vi "Draw.vi"(8 "error in (no error)":errorcluster, 10 "2D Picture in":picture, 11 "RoundRectangle in":refnum<class "RoundRectangle.lvclass">) -> (0 "error out":errorcluster, 2 "2D Picture out":picture, 3 "RoundRectangle out":refnum<class "RoundRectangle.lvclass">)   [LabVIEW 2021, in "Picture2D.lvlib" / "RoundRectangle.lvclass"]
uses:
  RoundRectangle.lvclass
  RoundRectangle.lvclass/RoundRectangle.ctl
  Rectangle/Rectangle.lvclass
  Color/Color.lvclass
  C:/Users/daal/OneDrive/LabVIEW/Class/Picture2D/Rectangle/Rectangle.lvclass
  C:/Users/daal/OneDrive/LabVIEW/Class/Picture2D/Polygone/Polygone.lvclass
  C:/Users/daal/OneDrive/LabVIEW/Class/Picture2D/Shape/Shape.lvclass
  C:/Users/daal/OneDrive/LabVIEW/Class/Picture2D/Picture2D/Picture2D.lvclass
  C:/Users/daal/OneDrive/LabVIEW/Class/Picture2D/IDrawable/IDrawable.lvclass
  C:/Users/daal/OneDrive/LabVIEW/Class/Picture2D/IMovable/IMovable.lvclass
  C:/Users/daal/OneDrive/LabVIEW/Class/Picture2D/IRotatable/IRotatable.lvclass
  C:/Users/daal/OneDrive/LabVIEW/Class/Picture2D/IScalable/IScalable.lvclass
  C:/Users/daal/OneDrive/LabVIEW/Class/Picture2D/RoundRectangle/RoundRectangle.lvclass
  Pen/Pen.lvclass
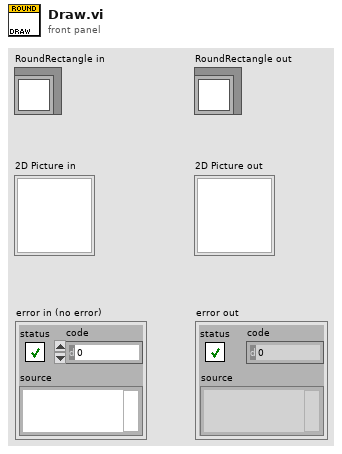
[diagram p1: front panel]
types:
  T1 = cluster{"left":i16, "top":i16, "right":i16, "bottom":i16}
  T2 = cluster{"Width":u16, "Style":enum32{"Solid", "Dash", "Dot", "DashDot", "DashDotDot"}}
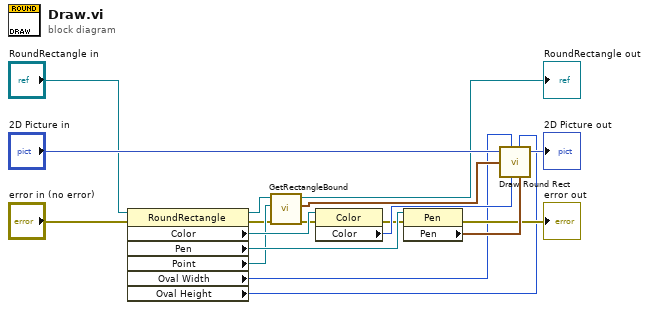
[diagram p0: block diagram]
diagram:
  n1 = property class="RoundRectangle"(reference="RoundRectangle in", error in="error in (no error)") -> (reference out=w4:refnum<class "RoundRectangle.lvclass">, error out=w9:errorcluster, "Color"=w15:refnum<class "Color.lvclass">, "Pen"=w13:refnum<class "Pen.lvclass">, "Point"=w11:refnum<class "Point.lvclass">, "Oval Width"=w2:i16, "Oval Height"=w1:i16)
  n2 = call "GetRectangleBound.vi"("error in (no error)"=w9, "Point"=w11, "Rectangle in"=w4) -> ("error out"=w8:errorcluster, "rect"=w10:T1, "Rectangle out"=→"RoundRectangle out":refnum<class "RoundRectangle.lvclass">)  [unwired: 6 in]
  n3 = property class="Color"(reference=w15, error in=w8) -> (error out=w7:errorcluster, "Color"=w14:u32)  [unwired: 1 out]
  n4 = property class="Pen"(reference=w13, error in=w7) -> (error out=→"error out":errorcluster, "Pen"=w12:T2)  [unwired: 1 out]
  n5 = call <vilib>:"Draw Round Rect.vi"("picture"="2D Picture in", "oval width"=w2, "rect"=w10, "color(black)"=w14, "oval height"=w1, "pen"=w12) -> ("new picture"=→"2D Picture out":picture)  [unwired: 3 in]
